vi "Write Array of Conflict Zones.vi"(10 "Array of Conflict Zones":T1[](array[typedef]) caption="Conflict Zones (unit in mm)", 11 "VacuumLines in":refnum<class "VacuumLines.lvclass">) -> (3 "VacuumLines out":refnum<class "VacuumLines.lvclass">)   [LabVIEW 2016, in "Hardware.lvlib" / "VacuumLine.lvlib" / "VacuumLines.lvclass"]
uses:
  <userlib>/Common Components/Hardware/Abstract System/VacuumLine/VacuumLines/VacuumLines.lvclass
  <userlib>/Common Components/Hardware/Abstract System/VacuumLine/VacuumLines/Conflict Zone.ctl
  <userlib>/Common Components/Hardware/Abstract System/VacuumLine/VacuumLines/VacuumLines.lvclass/VacuumLines.ctl
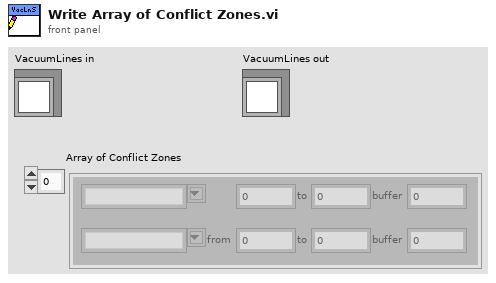
[diagram p1: front panel]
types:
  T1 = typedef "Hardware.lvlib/VacuumLine.lvlib/VacuumLines.lvclass/Conflict Zone.ctl" = cluster{"1":cluster{"Label":string, "from":dbl, "to":dbl, "buffer":dbl}, "2":cluster{"Label":string, "from":dbl, "to":dbl, "buffer":dbl}}
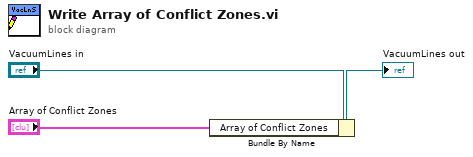
[diagram p0: block diagram]
diagram:
  n1 = Bundle By Name(cluster="VacuumLines in", "Array of Conflict Zones"="Array of Conflict Zones") -> (→"VacuumLines out":refnum<class "VacuumLines.lvclass">)
